vi "ABB norma 5000 Query Measurements.vi"(6 "Phase":i32[](array[numeric]) min=-1 max=64 step=1, 8 "error in (no error)":errorcluster, 9 "Modifier":i32[](array[ring]) items=["None", "Minimum", "Maximum", "Integral Positive", "Integral Negative", "Integral"], 10 "Measurement":i32[](array[ring]) items=["Voltage True RMS", "Voltage Mean", "Voltage Rectified Mean ", "Voltage Peak-To-Peak ", "Voltage Highest Value ", "Voltage Lowest Value ", "Voltage Crest Factor", "Voltage Absolute Phase", "Voltage True RMS Phase-To-Phase", "Voltage Harmonic", "Voltage TRMS Phase-To-Phase Harmonic", "Voltage Form Factor", "Voltage Harmonic Content", "Voltage Fundamental Content", "Voltage THD", "Current True RMS", "Current Mean", "Current Rectified Mean ", "Current Peak-To-Peak ", "Current Highest Value ", "Current Lowest Value", "Current Crest Factor", "Current Absolute Phase", "Current Harmonic", "Current Form Factor", "Current Harmonic Content", "Current Fundamental Content", "Current THD", "Power Active", "Power Apparent", "Power Reactive", "Power Factor", "Power Active Harmonic", "Power Apparent Harmonic", "Power Reactive Harmonic", "Power Factor Harmonic", "Power Corrected", "Phase", "Phase Harmonic", "Impedance", "Resistance Serial", "Resistance Parallel", "Reactance Serial", "Reactance Parallel", "Impedance Harmonic", "Resistance Serial Harmonic", "Resistance Parallel Harmonic", "Reactance Serial Harmonic", "Reactance Parallel Harmonic", "Frequency", "Averaging Interval", "Shaft Torque", "Rotational Speed", "Mechanical Power", "Rotational Asynchronousity", "Motor Efficiency", "Raw Process Input Value ", "Voltage Mean Phase-To-Phase", "Voltage Rectified Mean Phase-To-Phase", "Voltage Form Factor Phase-To-Phase", "Averaging Interval Relative Timestamp", "Electrical Efficiency", "Electrical Efficiency Harmonic", "True RMS Voltage Without DC", "True RMS Current Without DC"], 11 "VISA session":refnum<visa-resource-name>) -> (0 "error out":errorcluster, 2 "Data":dbl[](array[numeric]) format="%.2f", 3 "dup VISA session":refnum<visa-resource-name>)   [LabVIEW 2017]
doc: "This VI queries last valid measurements. No measurement is initiated with this function.\n\nNote:\n(1) All measured values returned by this function come from the same averaging interval."
panel:
  # "Starting from version 1.2.1 the numbering of function changed.\nNO compatibility with previous version!!!!!\nSee description of control."
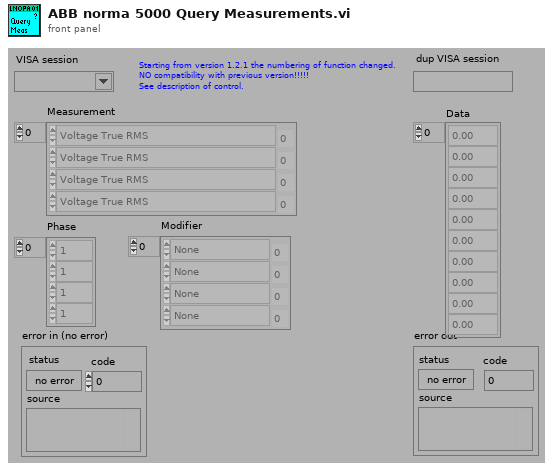
[diagram p1: front panel]
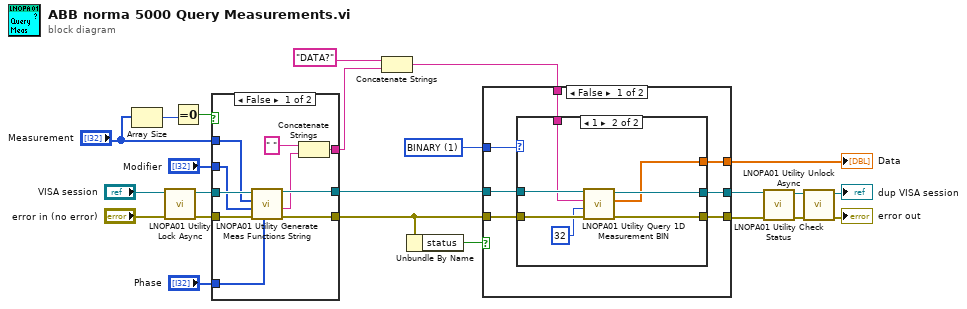
[diagram p0: block diagram]
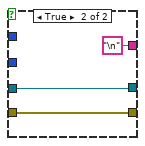
[diagram p2: hidden frame]
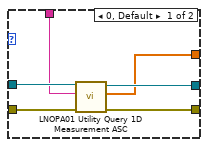
[diagram p3: hidden frame]
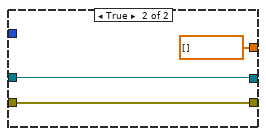
[diagram p4: hidden frame]
diagram:
  w21 = 1 items=["ASCII", "BINARY"] ("Format")
  n1 = Array Size(array="Measurement") -> (size(s)=w14:i32)
  n2 = call "LNOPA01 Utility Lock Async.vi"("error in (no error)"="error in (no error)", "VISA session"="VISA session") -> ("error out"=w6:errorcluster, "dup VISA session"=w5:refnum<visa-resource-name>)  [unwired: 8 in]
  n3 = Equal To 0?(x=w14) -> (x = 0?=w13:bool)
  n4 = case shown="False" w13 {
    tunnel: [w33 w35] -> w18
    tunnel: w5 -> [w32 w36]
    tunnel: w6 -> [w24 w35]
    tunnel: [w31 w36] -> w17
    tunnel: "Phase" -> [w30 _]
    tunnel: "Measurement" -> [w29 _]
    tunnel: "Modifier" -> [w28 _]
    tunnel: [w25 "\n"] -> w10
    frame False {
      n5 = call "LNOPA01 Utility Generate Meas Functions String.vi"("Phase"=w30, "error in (no error)"=w24, "Modifier"=w28, "Measurement"=w29, "VISA session"=w32) -> ("error out"=w33:errorcluster, "String"=w26:string, "dup VISA session"=w31:refnum<visa-resource-name>)  [unwired: 4 in]
      n6 = Concatenate Strings(" " ("Substring"), w26) -> (w25:string)
    }
    frame True {
    }
  }
  n7 = Concatenate Strings("DATA?" ("Command"), w10) -> (w16:string)
  n8 = Unbundle By Name(w18) -> ("status"=w23:bool)
  n9 = case shown="False" w23 {
    tunnel: w18 -> [w43 w57]
    tunnel: w17 -> [w42 w58]
    tunnel: w16 -> [w41 _]
    tunnel: [w40 w58] -> w20
    tunnel: [w39 w57] -> w19
    tunnel: [w38 dbl[] [] ("Data")] -> w22
    tunnel: w21 -> [w37 _]
    frame False {
      n10 = case shown="1" w37 {
        tunnel: w43 -> [w44 w56]
        tunnel: w42 -> [w49 w55]
        tunnel: w41 -> [w48 w54]
        tunnel: [w47 w53] -> w40
        tunnel: [w46 w52] -> w39
        tunnel: [w45 w51] -> w38
        frame 0, Default {
          n11 = call "LNOPA01 Utility Query 1D Measurement ASC.vi"("error in (no error)"=w44, "Command"=w48, "VISA session"=w49) -> ("error out"=w46:errorcluster, "Data"=w45:dbl[], "dup VISA session"=w47:refnum<visa-resource-name>)  [unwired: 5 in, 1 out]
        }
        frame 1 {
          n12 = call "LNOPA01 Utility Query 1D Measurement BIN.vi"("error in (no error)"=w56, "Width"=32, "Command"=w54, "VISA session"=w55) -> ("error out"=w52:errorcluster, "Data"=w51:dbl[], "dup VISA session"=w53:refnum<visa-resource-name>)  [unwired: 4 in, 1 out]
        }
      }
    }
    frame True {
    }
  }
  "Data" <- w22
  n13 = call "LNOPA01 Utility Check Status.vi"("error in (no error)"=w19, "VISA session"=w20) -> ("error out"=w3:errorcluster, "dup VISA session"=w4:refnum<visa-resource-name>)  [unwired: 8 in]
  n14 = call "LNOPA01 Utility Unlock Async.vi"("error in (no error)"=w3, "VISA session"=w4) -> ("error out"=→"error out":errorcluster, "dup VISA session"=→"dup VISA session":refnum<visa-resource-name>)  [unwired: 8 in]
